vi "DS345.set frequency.vi"(0 "i ref in":refnum<vi>, 2 "frequency [Hz]":dbl=0.01 min=0.01 max=10.0 format="%.3f", 5 "error in (no error)":errorcluster) -> (14 "i ref out":refnum<vi>, 19 "error out":errorcluster)   [LabVIEW 2014, in "DS345.lvlib"]
doc: "sets the frequency of the device"
uses:
  DS345.lvlib
  CS_Core/CSApplicationBaseClasses/AFGBase/AFGBase.directionType.ctl
  CS_Core/CSApplicationBaseClasses/AFGBase/AFGBase.serviceType.ctl
  CSlibraries/UtilityLib/UtilityLib.valueStatus.ctl
  CS_Core/CSApplicationBaseClasses/DeviceBase/DeviceBase.deviceState.ctl
  CS_Core/CSSystem/CoreDefs/CoreDefs.error_type.ctl
  instr.lib/Ds345/DS345Driver.lvlib
  CS_Core/CSSystem/CoreLib/CoreLib.lvlib
  CS_Core/CSApplicationBaseClasses/AFGBase/AFGBase.lvlib
  CS_Core/CSApplicationBaseClasses/DeviceBase/DeviceBase.lvlib
  CSlibraries/UtilityLib/UtilityLib.lvlib
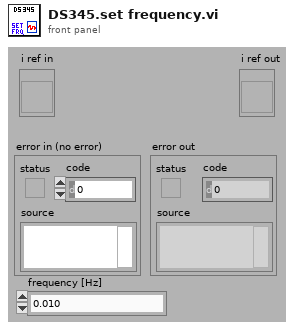
[diagram p1: front panel]
types:
  T1 = typedef "AFGBase.lvlib/AFGBase.serviceType.ctl" = enum16{"frequency", "amplitude", "phase", "DCOffset", "enableOutput", "trigger", "waveformType"}
  T2 = typedef "AFGBase.lvlib/AFGBase.directionType.ctl" = enum16{"unknown", "update actual value", "update nominal value", "update both"}
  T3 = typedef "UtilityLib.lvlib/UtilityLib.valueStatus.ctl" = enum16{"no info available", "stand by/off", "on", "warning", "alarm/malfunction", "not implemented", "user action required", "important information", "system default", "control default", "indicator default", "button default"}
  T4 = typedef "CoreDefs.error_type.ctl" = enum16{"no error", "can't load process", "can't unload process", "process does not exist", "can't install process", "can't remove process", "unknown function", "time out", "can't execute function", "duplicate queue name", "super not found", "caller queue invalid", "can't ping process", "unknown error", "VISA Error", "VISA timeout", "GPIB timeout", "GPIB error", "communication error", "data type mismatch", "can't read data from OPC server", "can't write data to OPC server", "OET error", "function not implemented", "process already exists", "invalid Shared Variable name", "error writing Shared Variable", "error reading Shared Variable", "invalid client name", "corrupt database", "unknown class", "call not authorized", "parameter out of range", "OET timeout: can't get data to modify", "invalid queue name", "requested operation incompatible with current state", "event undefined", "event disabled", "state undefined", "caller is not a friend", "EventBuilder: bad eventID", "EventBuilder: no DAQ devices", "a thread must not stop itself", "UNUSED ELEMENT4", "DiscArchiver: eventData incomplete", "DiscArchiver: eventData does not belong to run", "DiscArchiver: can't open file", "DiscArchiver: can't write to file", "DiscArchiver: available disc space low", "can't acquire semaphore", "error reading data from database", "notifier object is not existing", "can't register process", "can't unregister process", "illegal event type", "object disabled", "object already exists", "can't change state", "Instrument not found", "no connection to remote node", "invalid reference", "N/A", "UNUSED ELEMENT 1", "element not found", "illegal TCP/IP connection detected", "object does not exist", "invalid access ID", "unknown CS system", "invalid privilige", "unsupported data type", "unsupported server type", "IO server already exists", "Shared Variable already exists"}
  T5 = typedef "DeviceBase.lvlib/DeviceBase.deviceState.ctl" = i16
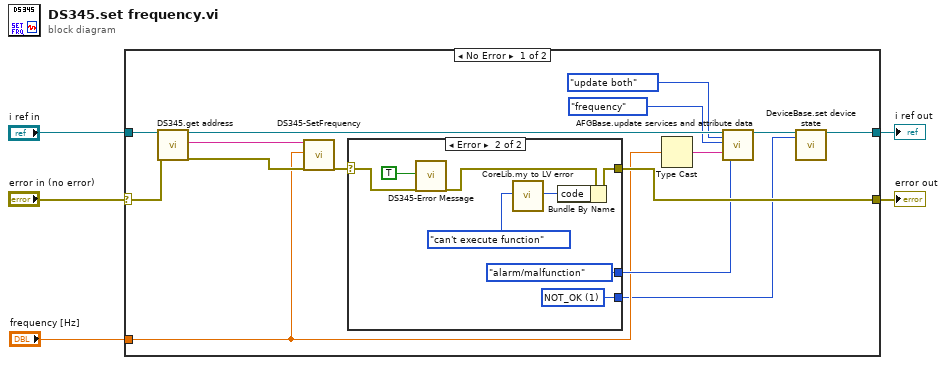
[diagram p0: block diagram]
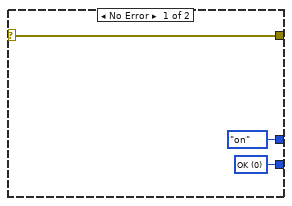
[diagram p2: hidden frame]
diagram:
  n1 = case shown="No Error" "error in (no error)" {
    selector: "error in (no error)" -> [w16 w32]
    tunnel: [w14 w32] -> w5
    tunnel: "i ref in" -> [w20 w33]
    tunnel: "frequency [Hz]" -> [w7 _]
    tunnel: [w12 w33] -> w2
    frame No Error {
      n2 = call "DS345.get address.vi"("i ref in"=w20, "error in (no error)"=w16) -> ("i ref out"=w15:refnum<vi>, "address"=w18:string, "error out"=w19:errorcluster)  [unwired: 15 in]
      n3 = call "DS345-SetFrequency.vi"("address string"=w18, "frequency [Hz]"=w7, "error in (no error)"=w19) -> ("error out"=w17:errorcluster)  [unwired: 15 in, 1 out]
      n4 = case shown="Error" w17 {
        selector: w17 -> [w23 w28]
        tunnel: [w23 w31] -> w14
        tunnel: [UtilityLib.valueStatus."on" ("quality") UtilityLib.valueStatus."alarm/malfunction" ("quality")] -> w8
        tunnel: [w21 w24] -> w6
        frame No Error {
          w21 = T5 0 items=["ERROR"=-1, "OK"=0, "NOT_OK"=1] ("deviceState")
        }
        frame Error {
          w24 = T5 1 items=["ERROR"=-1, "OK"=0, "NOT_OK"=1] ("deviceState")
          n5 = call "DS345-Error Message.vi"("addMessageToSource"=TRUE ("add message to source"), "error in (no error)"=w28) -> ("error out"=w27:errorcluster)  [unwired: 14 in, 3 out]
          n6 = call "CoreLib.my to LV error.vi"("ErrorTypes"=CoreDefs.error_type."can't execute function") -> ("LV error code"=w30:i32)  [unwired: 17 in, 1 out]
          n7 = Bundle By Name(cluster=w27, "code"=w30) -> (w31:errorcluster)
        }
      }
      n8 = Type Cast(x=w7) -> (*(type *) &x=w9:string)  [unwired: 1 in]
      n9 = call "AFGBase.update services and attribute data.vi"("i ref in"=w15, "direction"=AFGBase.directionType."update both", "service"=AFGBase.serviceType."frequency", "value"=w9, "quality"=w8) -> ("i ref out"=w13:refnum<vi>)  [unwired: 12 in, 2 out]
      n10 = call "DeviceBase.set device state.vi"("i ref in"=w13, "deviceState"=w6) -> ("i ref out"=w12:refnum<vi>)  [unwired: 15 in, 2 out]
    }
    frame Error {
    }
  }
  "error out" <- w5
  "i ref out" <- w2
